vi "valve_VCH.vi"(6 "Parameters table VCH":u32[](array[numeric])=[0, 10000, 0, 0, 0, 0, 0, 5000, 1000, 0, 2], 7 "Alarm":bool[](array[boolean])=[FALSE, FALSE], 9 "ZB01 (F)":bool, 10 "XB24 (F)":bool, 11 "Z_control":T5={"Z_HSw"=1, "Z_HSetState"=enum."on (closed)", "Z_ASetState"=enum."on (closed)", "Z_DSetState"=enum."on (closed)"}) -> (2 "YB":bool[](array[boolean]), 3 "Z_State":T1={"Z_Source"=enum."local disabled", "Z_SetState"=enum."initialization", "Z_State"=enum."initialization", "Z_State_T"=0, "ZM_State"=enum."initialization", "ZM_State_T"=0, "ALR  L1"=FALSE, "ALR  L2"=FALSE, "HH_run"=0}, 4 "ZM_State_next":u32, 5 "ALR_ON":bool[](array[boolean]))   [LabVIEW 2019, in "Valves.lvlib"]
uses:
  Valves.lvlib
  ctl/Z_State_VCH.ctl
  Heating/ctl/Y_source.ctl
  Heating/Heating.lvlib
  ctl/Z.ctl
  ctl/ZM_State_VCH.ctl
  ctl/Z_control_VCH.ctl
panel:
  # "Alarm_L1"
  # "Alarm_L2"
  # "T_valve_open_state"
  # "T_restart_delay"
  # "T_valve_open"
  # "T_valve_close"
  # "T_little_pause"
  # "T_start_delay"
  # "T_stop_delay"
  # "T_big_pause"
  # "N_repeat"
  # "T_check"
  # "TsStop"
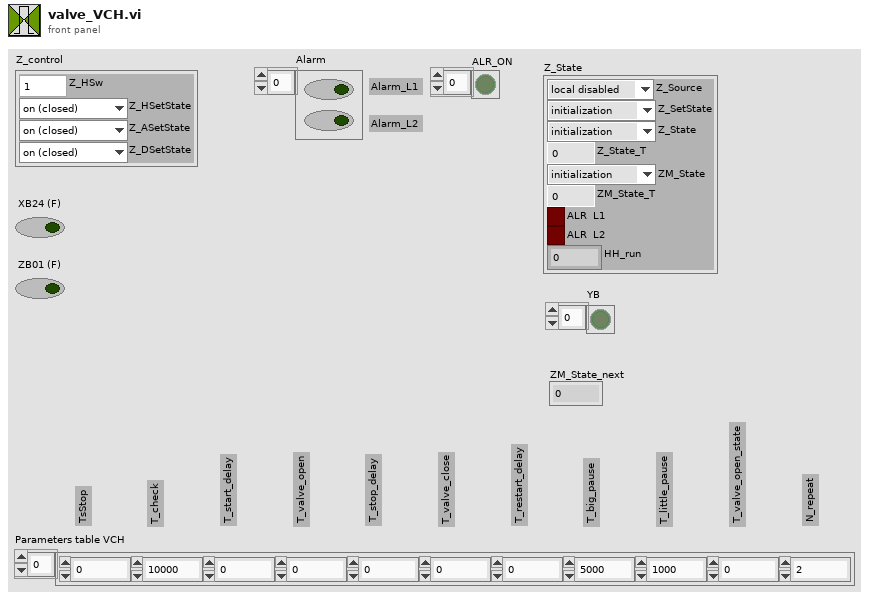
[diagram p1: front panel]
types:
  T1 = typedef "Valves.lvlib/Z.ctl" = cluster{"Z_Source":T2, "Z_SetState":T3, "Z_State":T3, "Z_State_T":u32, "ZM_State":T4, "ZM_State_T":u32, "ALR  L1":bool, "ALR  L2":bool, "HH_run":i32}
  T2 = typedef "Heating.lvlib/Y_source.ctl" = enum8{"initialize", "local disabled", "local hand", "hand", "auto", "dist"}
  T3 = typedef "Valves.lvlib/Z_State_VCH.ctl" = enum8{"initialization", "alarm", "disabled", "not ready", "closed ready", "reserv", "reserv1", "reserv2", "reserv3", "check", "on min", "open", "on (closed)"}
  T4 = typedef "Valves.lvlib/ZM_State_VCH.ctl" = enum8{"initialization", "closed", "big_pause", "little_pause", "open", "close_cmd"}
  T5 = typedef "Valves.lvlib/Z_control_VCH.ctl" = cluster{"Z_HSw":u8, "Z_HSetState":T3, "Z_ASetState":T3, "Z_DSetState":T3}
  T6 = cluster{"Z_Source":T2, "Z_State":T3, "ZM_State":T4}
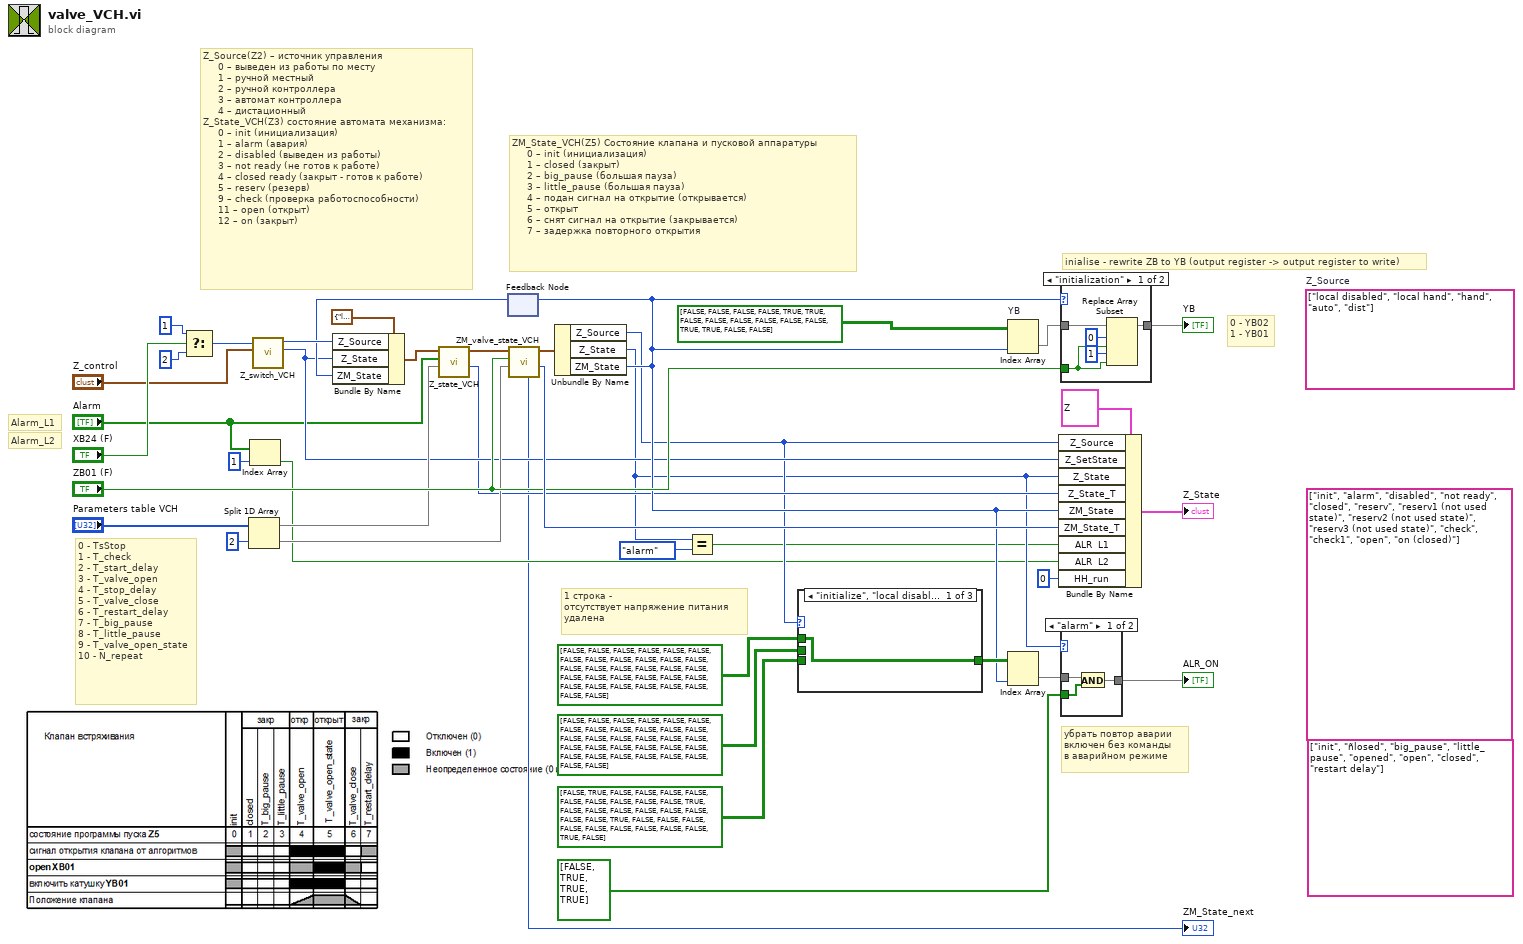
[diagram p0: block diagram]
diagram:
  (unwired) string[] ["init", "alarm", "disabled", "not ready", "closed", "reserv", "reserv1 (not used state)", "reserv2 (not used state)", "reserv3 (not used state)", "check", "check1", "open", "on (closed)"]
  (unwired) string[] ["local disabled", "local hand", "hand", "auto", "dist"]  # Z_Source
  (unwired) string[] ["init", "ñlosed", "big_pause", "little_pause", "opened", "open", "closed", "restart delay"]
  # "Alarm_L2"
  # "Alarm_L1"
  # "inialise - rewrite ZB to YB (output register -> output register to write)"
  # "0 - YB02\n1 - YB01"
  # "1 строка - \nотсутствует напряжение питания\nудалена"
  # "убрать повтор аварии\nвключен без команды\nв аварийном режиме"
  # "0 - TsStop\n1 - T_check\n2 - T_start_delay\n3 - T_valve_open\n4 - T_stop_delay\n5 - T_valve_close\n6 - T_restart_delay\n7 - T_big_pause\n8 - T_little_pause\n9 - T_valve_open_state\n10 - N_repeat"
  # "Z_Source(Z2) – источник управления\n     0 – выведен из работы по месту\n     1 – ручной местный\n     2 – ручной контроллера\n     3 – автомат контроллера\n     4 – дистационный\nZ_State_VCH(Z3) состояние автомата механизма:\n     0 – init (инициализация)\n     1 – alarm (авария)\n     2 – disabled (выведен из работы)\n     3 – not ready (не готов к работе)\n     4 – closed ready (закрыт - готов к работе)\n     5 – reserv (резерв)\n     9 – check (проверка работоспособности)\n     11 – open (открыт)\n     12 – on (закрыт)"
  # "ZM_State_VCH(Z5) Состояние клапана и пусковой аппаратуры\n     0 – init (инициализация)\n     1 – сlosed (закрыт)\n     2 – big_pause (большая пауза)\n     3 – little_pause (большая пауза)\n     4 – подан сигнал на открытие (открывается)\n     5 – открыт\n     6 – снят сигнал на открытие (закрывается)\n     7 – задержка повторного открытия"
  n1 = Select(t=u32 1, s="XB24 (F)", f=u32 2) -> (s? t:f=w38:u32)
  n2 = Split 1D Array(array="Parameters table VCH", index=2) -> (first subarray=w20:u32[], second subarray=w19:u32[])
  n3 = Index Array(array="Alarm", index=1) -> (element=w4:bool)
  n4 = call "Z_switch_VCH.vi"("Z"="Z_control", "Z_LSw (2-auto)"=w38) -> ("Z_SetState"=w13:T3, "Z_Source"=w27:T2)  [unwired: 8 in]
  n5 = feedback #1() -> (w25:T4)  [unwired: 1 in]
  n6 = Bundle By Name(cluster=T6 {"Z_Source"=enum."local disabled", "Z_State"=enum."initialization", "ZM_State"=enum."initialization"} ("Z_In"), "Z_Source"=w27, "Z_State"=w13, "ZM_State"=w25) -> (w26:T6)
  n7 = call "Z_state_VCH.vi"("Time"=w20, "Alarm"="Alarm", "Z_In"=w26) -> ("t"=w12:u32, "Z_Out"=w16:T6)  [unwired: 7 in]
  n8 = call "ZM_valve_state_VCH.vi"("Parameters table MVCH"=w19, "ZB01"="ZB01 (F)", "Z_In"=w16) -> ("t"=w28:u32, "Z_Out"=w18:T6, "ZM_State_next"=→"ZM_State_next":u32)  [unwired: 6 in]
  n9 = Unbundle By Name(w18) -> ("Z_Source"=w10:T2, "Z_State"=w9:T3, "ZM_State"=w14:T4)
  n10 = feedback-in #1(w14) -> ()
  n11 = Equal?(x=w9, y=Z_State_VCH."alarm") -> (x = y?=w7:bool)
  n12 = case shown="\"initialize\", \"local disabled\"" w10 {
    tunnel: bool[][] [[FALSE, FALSE, FALSE, FALSE, FALSE, FALSE, FALSE, FALSE], [FALSE, FALSE, FALSE, FALSE, FALSE, FALSE, FALSE, FALSE], [FALSE, FALSE, FALSE, FALSE, FALSE, FALSE, FALSE, FALSE], [FALSE, FALSE, FALSE, FALSE, FALSE, FALSE, FALSE, FALSE]] ("Array") -> [w42 _ _]
    tunnel: bool[][] [[FALSE, FALSE, FALSE, FALSE, FALSE, FALSE, FALSE, FALSE], [FALSE, FALSE, FALSE, FALSE, FALSE, FALSE, FALSE, FALSE], [FALSE, FALSE, FALSE, FALSE, FALSE, FALSE, FALSE, FALSE], [FALSE, FALSE, FALSE, FALSE, FALSE, FALSE, FALSE, FALSE]] ("Array 2") -> [_ w43 _]
    tunnel: bool[][] [[FALSE, TRUE, FALSE, FALSE, FALSE, FALSE, FALSE, FALSE], [FALSE, FALSE, FALSE, TRUE, FALSE, FALSE, FALSE, FALSE], [FALSE, FALSE, FALSE, FALSE, TRUE, FALSE, FALSE, FALSE], [FALSE, FALSE, FALSE, FALSE, FALSE, FALSE, TRUE, FALSE]] ("Array 3") -> [_ _ w44]
    tunnel: [w42 w43 w44] -> w34
    frame "initialize", "local disabled" {
    }
    frame "local hand" {
    }
    frame "hand", Default {
    }
  }
  n13 = Index Array "YB"(array=bool[][] [[FALSE, FALSE, FALSE, FALSE, TRUE, TRUE, FALSE, FALSE], [FALSE, FALSE, FALSE, FALSE, TRUE, TRUE, FALSE, FALSE]] ("Array 5"), index (col)=w14) -> (element=w30:bool[])  [unwired: 1 in]
  n14 = Index Array(array=w34, index (col)=w14) -> (element=w32:bool[])  [unwired: 1 in]
  n15 = Bundle By Name(cluster=T1 {"Z_Source"=enum."local disabled", "Z_SetState"=enum."initialization", "Z_State"=enum."initialization", "Z_State_T"=0, "ZM_State"=enum."initialization", "ZM_State_T"=0, "ALR  L1"=FALSE, "ALR  L2"=FALSE, "HH_run"=0} ("Z"), "Z_Source"=w10, "Z_SetState"=w13, "Z_State"=w9, "Z_State_T"=w12, "ZM_State"=w14, "ZM_State_T"=w28, "ALR  L1"=w7, "ALR  L2"=w4, "HH_run"=0) -> (→"Z_State":T1)
  n16 = case shown="\"initialization\"" w14 {
    tunnel: w30 -> [w49 w50]
    tunnel: [w46 w50] -> w29
    tunnel: "ZB01 (F)" -> [w45 _]
    frame "initialization" {
      n17 = Replace Array Subset(array=w49, new element #1=w45, index #1=0 ("index"), new element #2=w45, index #2=1 ("index")) -> (w46:bool[])
    }
    frame "closed", Default {
    }
  }
  "YB" <- w29
  n18 = case shown="\"alarm\"" w9 {
    tunnel: bool[] [FALSE, TRUE, TRUE, TRUE] ("Array 4") -> [w52 _]
    tunnel: w32 -> [w53 w54]
    tunnel: [w51 w54] -> w31
    frame "alarm" {
      n19 = And(x=w53, y=w52) -> (x .and. y?=w51:bool[])
    }
    frame "disabled", Default {
    }
  }
  "ALR_ON" <- w31
